vi "Fire.vi"(8 "error in (no error)":errorcluster, 11 "?":T1) -> (0 "error out":errorcluster)   [LabVIEW 2013]
uses:
  ShooterCmds.ctl
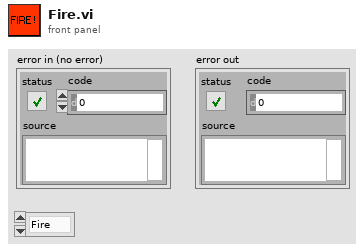
[diagram p1: front panel]
types:
  T1 = typedef "ShooterCmds.ctl" = enum16{"Fire", "Lob", "Retract"}
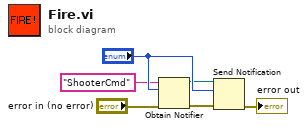
[diagram p0: block diagram]
diagram:
  n1 = Obtain Notifier(name (unnamed)="ShooterCmd", notification data type="?", error in (no error)="error in (no error)") -> (notifier out=w4:refnum<notifier>, error out=w6:errorcluster)  [unwired: 1 in, 1 out]
  n2 = Send Notification(notification="?", notifier=w4, error in (no error)=w6) -> (error out=→"error out":errorcluster)  [unwired: 1 out]
